vi "QuadEncCalcSGL_gen.vi"(0 "AbsPosition":i32, 5 "RevPosition":i32, 9 "input valid":bool=TRUE, 11 "RevPerPulse":sgl, 12 "dTPerSec":sgl) -> (4 "Revolutions":sgl, 6 "RevPerSec":sgl, 8 "Theta":sgl, 10 "output valid":bool, 14 "feedback signals":cluster{"ready for input":bool}, 15 "RadPerSec":sgl)   [LabVIEW 2015]
doc: "This VI is created by the NI LabVIEW 2015 FPGA IP Builder.\n\nProject: QuadEnc_dev.lvproj\nTarget: FPGA Target (sbRIO-9607)/IP Builder\nBuild Specification: QuadEncCalcSGL_src\nDirectives Item: QuadEncCalcSGL_src\nTop-Level VI: C:\\perforce\\Sales\\projects\\Energy\\InverterIP\\QuadratureEncoder\\IPBuilder\\QuadEncCalcSGL_src.vi\n\nQuick Device Utilization Estimate\n--------------------------------------------\nSlice Registers: 1.1% (1188 out of 106400)\nSlice LUTs: 5.8% (3064 out of 53200)\nDSP48s: 3.6% (8 out of 220)\nBlock RAMs: 0.0% (0 out of 280)\n\nQuick Performance Estimate\n--------------------------------------------\nClock rate (MHz): 49.53\nInitiation interval (cycles): 11\nPipeline type: Not pipelined\nMinimum latency: 10\nMaximum latency: 10"
uses:
  <vilib>/rvi/IPIntegrationNode/IPINode_Typedef/niFpgaIPINodeSupportedFamilies.ctl
  <vilib>/rvi/IPIntegrationNode/IPINode_Utilities/niFpgaIPINodeSimCore.vi
  <vilib>/rvi/IPIntegrationNode/IPINode_Xnode/niFpgaIPINode.xnode
  QuadEncCalcSGL_gen Support/IPBlockSimFiles/xsim.dir/m032BACDA_topH/xsimkACD6C9554CFB4CFE8E98209D00B6F72E.dll
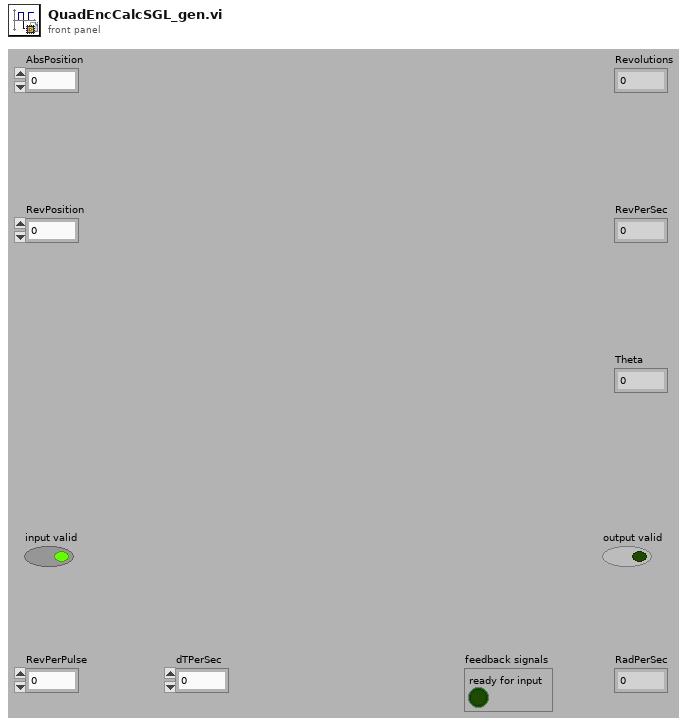
[diagram p1: front panel]
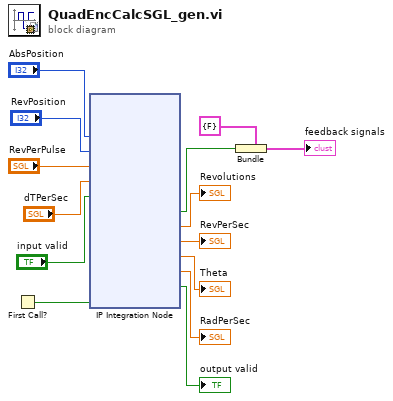
[diagram p0: block diagram]
diagram:
  n1 = First Call?() -> (First Call?: T/F=w14:bool)
  n2 = xnode "IP Integration Node"("p_11_AbsPosition"="AbsPosition", "p_10_RevPosition"="RevPosition", "p_8_RevPerPulse"="RevPerPulse", "p_6_dTPerSec"="dTPerSec", "input_valid"="input valid", "first_call"=w14) -> ("ready_for_input"=w11:bool, "p_3_Revolutions"=→"Revolutions":sgl, "p_2_RevPerSec"=→"RevPerSec":sgl, "p_1_Theta"=→"Theta":sgl, "p_0_RadPerSec"=→"RadPerSec":sgl, "output_valid"=→"output valid":bool)  [unwired: 2 in]
  n3 = Bundle ("Bundle_feedback")(cluster=cluster{"ready for input":bool} {"ready for input"=FALSE}, "ready for input"=w11) -> (→"feedback signals":cluster{"ready for input":bool})
